vi "reset_velocity.vi"() -> (3 "Numeric":dbl)   [LabVIEW 2022 SP3]
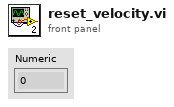
[diagram p1: front panel]
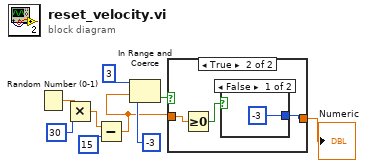
[diagram p0: block diagram]
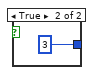
[diagram p3: hidden frame]
diagram:
  n1 = Random Number (0-1)() -> (number: 0 to 1=w9:dbl)
  n2 = Multiply(x=w9, y=30) -> (x*y=w7:dbl)
  n3 = Subtract(x=w7, y=15) -> (x-y=w2:dbl)
  n4 = In Range and Coerce(upper limit=3, x=w2, lower limit=-3) -> (In Range?=w5:bool)  [unwired: 1 out]
  n5 = case shown="True" w5 {
    tunnel: w2 -> [w10 w13]
    tunnel: [w10 w11] -> w1
    frame False {
    }
    frame True {
      n6 = Greater Or Equal To 0?(x=w13) -> (x >= 0?=w12:bool)
      n7 = case shown="False" w12 {
        tunnel: [-3 3] -> w11
        frame False {
        }
        frame True {
        }
      }
    }
  }
  "Numeric" <- w1
